vi "Configure Profile.vi"(7 "Pump ID (0:A)":T2, 8 "error in (no error)":errorcluster, 10 "Flow Parameters":T1={"Peak Flow (100 uL/s)"=100.0, "Starting Flow (0.1 uL/s)"=0.1, "Acceleration (500 uL/s^2)"=500.0, "Deceleration (500 uL/s^2)"=500.0}, 11 "VISA resource in":refnum<visa-resource-name>) -> (0 "error out":errorcluster, 3 "VISA resource out":refnum<visa-resource-name>)   [LabVIEW 2020, in "Global FIA milliGAT.lvlib"]
doc: "Configuration the motion settings:; initial flow rate, acceleration, deceleration, and max flow rate."
uses:
  <instrlib>/RxnRover/Global FIA milliGAT 3.14/Global FIA milliGAT.lvlib
  <instrlib>/RxnRover/Global FIA milliGAT 3.14/Public/Utility/Pump Address.ctl
  <instrlib>/RxnRover/Global FIA milliGAT 3.14/Private/Pump Parameter.ctl
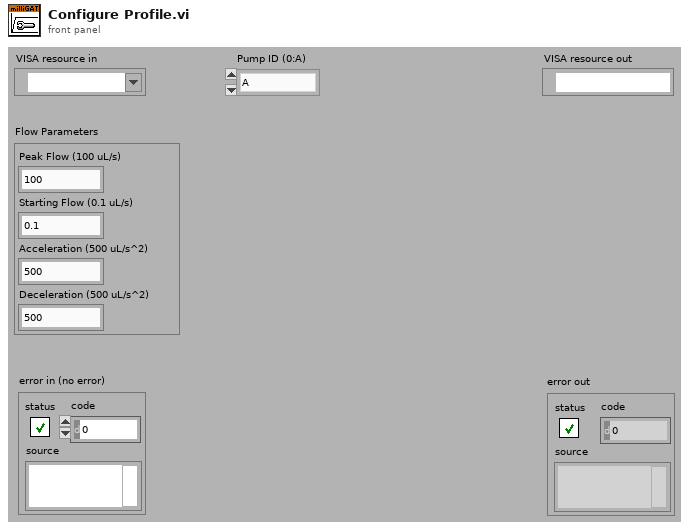
[diagram p1: front panel]
types:
  T1 = cluster{"Peak Flow (100 uL/s)":dbl, "Starting Flow (0.1 uL/s)":dbl, "Acceleration (500 uL/s^2)":dbl, "Deceleration (500 uL/s^2)":dbl}
  T2 = typedef "Global FIA milliGAT.lvlib/Pump Address.ctl" = enum16{"A", "B", "C", "D", "E", "F", "G", "H", "I", "J", "K", "L", "M", "N", "O", "P", "Q", "R", "S", "T", "U", "V", "W", "X", "Y", "Z", "a", "b", "c", "d", "e", "f", "g", "h", "i", "j", "k", "l", "m", "n", "o", "p", "q", "r", "s", "t", "u", "v", "w", "x", "y", "z", "0", "1", "2", "3", "4", "5", "6", "7", "8", "9"}
  T3 = typedef "Global FIA milliGAT.lvlib/Pump Parameter.ctl" = enum16{"Enabled", "EU", "EU Calibration Factor", "Fixed Asp or Disp", "Starting Position", "Starting Flow", "Peak Flow", "Flow Acceleration", "Flow Deceleration", "Session Volume", "Max Pressure", "Backlash (usteps)", "BL Calibration Factor", "BL Correction Enabled", "Min Flow", "Max Flow", "Min Acceleration", "Max Acceleration", "Service Volume", "Life Volume"}
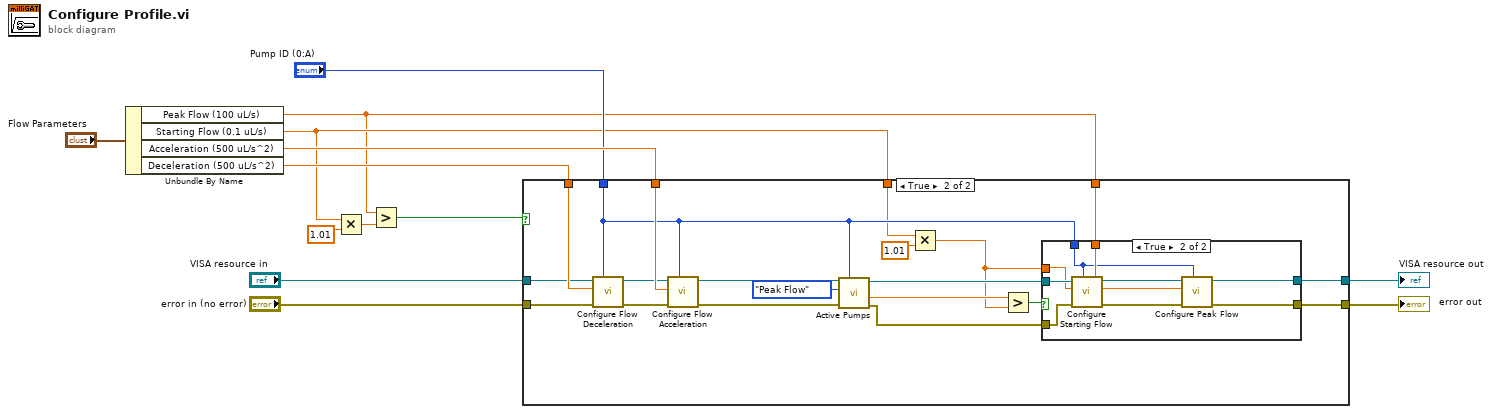
[diagram p0: block diagram]
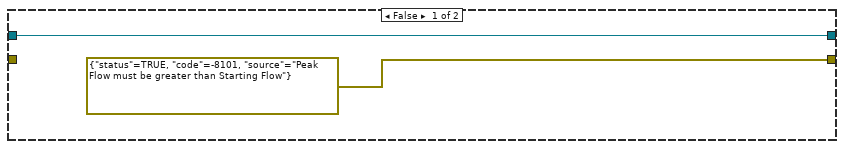
[diagram p2: hidden frame]
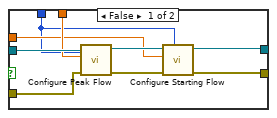
[diagram p3: hidden frame]
diagram:
  n1 = Unbundle By Name("Flow Parameters") -> ("Peak Flow (100 uL/s)"=w2:dbl, "Starting Flow (0.1 uL/s)"=w4:dbl, "Acceleration (500 uL/s^2)"=w11:dbl, "Deceleration (500 uL/s^2)"=w12:dbl)
  n2 = Multiply(x=w4, y=1.01) -> (x*y=w3:dbl)
  n3 = Greater?(x=w2, y=w3) -> (0:w1:bool)
  n4 = case shown="True" w1 {
    tunnel: w12 -> [_ w35]
    tunnel: w11 -> [_ w34]
    tunnel: "VISA resource in" -> [w15 w33]
    tunnel: [w15 w31] -> w9
    tunnel: [errorcluster {"status"=TRUE, "code"=-8101, "source"="Peak Flow must be greater than Starting Flow"} ("f") w30] -> w8
    tunnel: "error in (no error)" -> [_ w28]
    tunnel: "Pump ID (0:A)" -> [_ w24]
    tunnel: w4 -> [_ w21]
    tunnel: w2 -> [_ w27]
    frame False {
    }
    frame True {
      n5 = call <instrlib>:"Configure Flow Deceleration.vi"("Pump ID (0:A)"=w24, "error in (no error)"=w28, "Flow Deceleration  (500 uL/s^2)"=w35, "VISA resource in"=w33) -> ("error out"=w29:errorcluster, "VISA resource out"=w32:refnum<visa-resource-name>)  [unwired: 6 in]
      n6 = call <instrlib>:"Configure Flow Acceleration.vi"("Pump ID (0:A)"=w24, "error in (no error)"=w29, "Flow Acceleration  (500 uL/s^2)"=w34, "VISA resource in"=w32) -> ("error out"=w25:errorcluster, "VISA resource out"=w26:refnum<visa-resource-name>)  [unwired: 6 in]
      n7 = call <instrlib>:"Active Pumps.vi"("Pump ID (0:A)"=w24, "error in (no error)"=w25, "Parameter"=Pump_Parameter."Peak Flow", "VISA resource in"=w26) -> ("error out"=w17:errorcluster, "Value out"=w20:dbl, "VISA resource out"=w18:refnum<visa-resource-name>)  [unwired: 4 in, 1 out]
      n8 = Multiply(x=w21, y=1.01) -> (x*y=w16:dbl)
      n9 = Greater?(x=w20, y=w16) -> (0:w19:bool)
      n10 = case shown="True" w19 {
        tunnel: [w36 w52] -> w31
        tunnel: [w37 w51] -> w30
        tunnel: w27 -> [w43 w49]
        tunnel: w24 -> [w39 w48]
        tunnel: w18 -> [w44 w47]
        tunnel: w17 -> [w42 w46]
        tunnel: w16 -> [w40 w45]
        frame False {
          n11 = call <instrlib>:"Configure Peak Flow.vi"("Pump ID (0:A)"=w39, "error in (no error)"=w42, "Peak Flow (100 uL/s)"=w43, "VISA resource in"=w44) -> ("error out"=w38:errorcluster, "VISA resource out"=w41:refnum<visa-resource-name>)  [unwired: 6 in]
          n12 = call <instrlib>:"Configure Starting Flow.vi"("Pump ID (0:A)"=w39, "error in (no error)"=w38, "Starting Flow (0.1 uL/s)"=w40, "VISA resource in"=w41) -> ("error out"=w37:errorcluster, "VISA resource out"=w36:refnum<visa-resource-name>)  [unwired: 6 in]
        }
        frame True {
          n13 = call <instrlib>:"Configure Starting Flow.vi"("Pump ID (0:A)"=w48, "error in (no error)"=w46, "Starting Flow (0.1 uL/s)"=w45, "VISA resource in"=w47) -> ("error out"=w50:errorcluster, "VISA resource out"=w53:refnum<visa-resource-name>)  [unwired: 6 in]
          n14 = call <instrlib>:"Configure Peak Flow.vi"("Pump ID (0:A)"=w48, "error in (no error)"=w50, "Peak Flow (100 uL/s)"=w49, "VISA resource in"=w53) -> ("error out"=w51:errorcluster, "VISA resource out"=w52:refnum<visa-resource-name>)  [unwired: 6 in]
        }
      }
    }
  }
  "VISA resource out" <- w9
  "error out" <- w8
